vi "Main.vi"() -> ()   [LabVIEW 2025]
uses:
  Typedefs/MainState.ctl
  Typedefs/ConfigurationSettings.ctl
panel:
  in  "Reset":bool
  in  "Clear Data":bool
  in  "Configure":bool
  in  "Add Data":bool
  out "Waveform Chart":dbl[](graph)
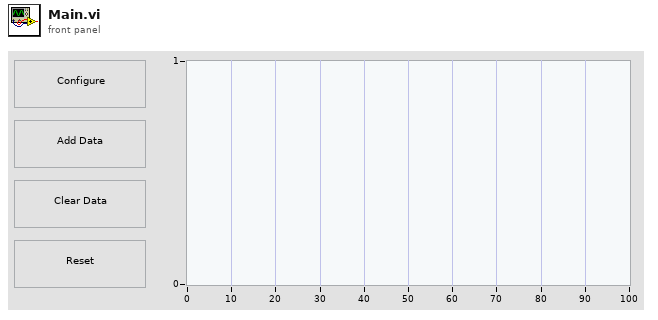
[diagram p1: front panel]
types:
  T1 = typedef "MainState.ctl" = enum16{"CONSTRUCT", "DESTRUCT", "WAITING_FOR_EVENT", "ADD_DATA", "CLEAR_DATA", "CONFIGURE", "RESET"}
  T2 = typedef "ConfigurationSettings.ctl" = cluster{"Plot.Line Width":u8, "Plot.Line Style":u8}
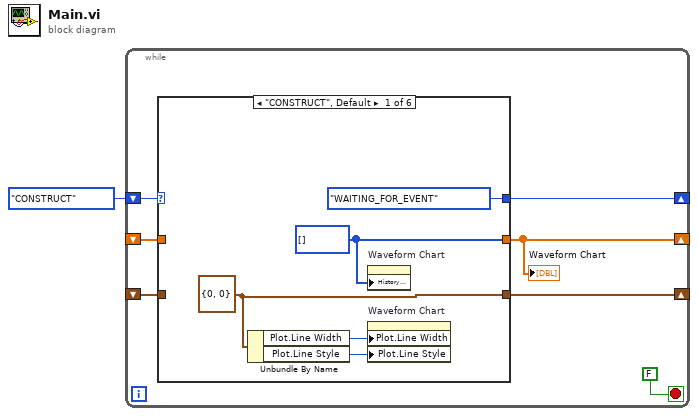
[diagram p0: block diagram]
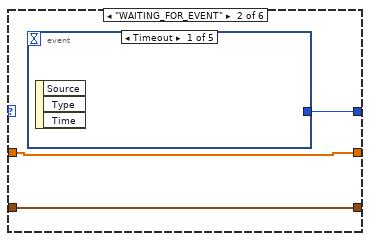
[diagram p2: hidden frame]
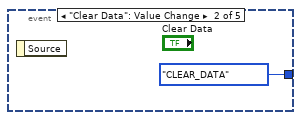
[diagram p3: hidden frame]
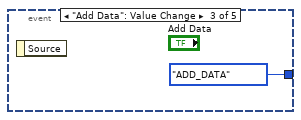
[diagram p4: hidden frame]
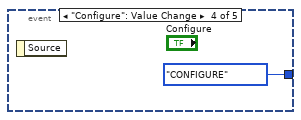
[diagram p5: hidden frame]
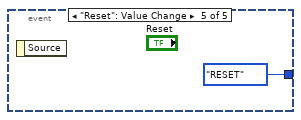
[diagram p6: hidden frame]
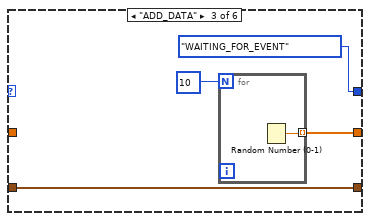
[diagram p7: hidden frame]
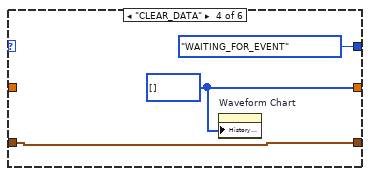
[diagram p8: hidden frame]
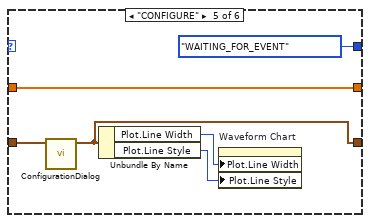
[diagram p9: hidden frame]
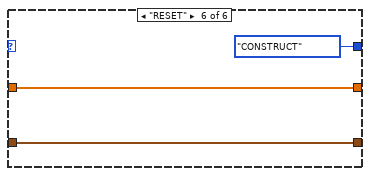
[diagram p10: hidden frame]
diagram:
  n1 = while {
    shift-right: [w6] -> _
    shift-left: MainState."CONSTRUCT" ("Main State") -> [w8]
    shift-right: [w7] -> _
    shift-left: _ -> [w5]
    shift-right: [w2] -> _
    shift-left: _ -> [w3]
    stop <- FALSE stop-if-true
    n2 = case shown="\"CONSTRUCT\", Default" w8 {
      tunnel: [w12 w15 w22 w27 w33 w36] -> w7
      tunnel: [MainState."WAITING_FOR_EVENT" ("Main State") w16 MainState."WAITING_FOR_EVENT" ("Main State") MainState."WAITING_FOR_EVENT" ("Main State") MainState."WAITING_FOR_EVENT" ("Main State") MainState."CONSTRUCT" ("Main State")] -> w6
      tunnel: w5 -> [_ w15 _ _ w33 w36]
      tunnel: w3 -> [_ w14 w21 w26 w32 w35]
      tunnel: [w11 w14 w21 w26 w31 w35] -> w2
      frame "CONSTRUCT", Default {
        w11 = T2 {"Plot.Line Width"=0, "Plot.Line Style"=0} ("ConfigurationSettings")
        w12 = i32[] []
        n3 = Unbundle By Name(w11) -> ("Plot.Line Width"=w10:u8, "Plot.Line Style"=w9:u8)
        n4 = property on="Waveform Chart" class="WFChart (strict)"("History Data"=w12) -> ()  [unwired: 2 in, 2 out]
        n5 = property on="Waveform Chart" class="WFChart (strict)"("Plot.Line Width"=w10, "Plot.Line Style"=w9) -> ()  [unwired: 2 in, 2 out]
      }
      frame "WAITING_FOR_EVENT" {
        n6 = event shown="[0] Timeout" {
          selector: _ -> [_ _ _ _ _]
          dyn-events: _ -> [_ _ _ _ _]
          timeout: _ -> [_ _ _ _ _]
          tunnel: [_ MainState."CLEAR_DATA" ("Main State") MainState."ADD_DATA" ("Main State") MainState."CONFIGURE" ("Main State") MainState."RESET" ("Main State")] -> w16
          event Timeout {
            n7 = event-data() -> ()  [unwired: 1 in, 3 out]
          }
          event "Clear Data": Value Change {
            n8 = event-data() -> ()  [unwired: 1 in, 1 out]
          }
          event "Add Data": Value Change {
            n9 = event-data() -> ()  [unwired: 1 in, 1 out]
          }
          event "Configure": Value Change {
            n10 = event-data() -> ()  [unwired: 1 in, 1 out]
          }
          event "Reset": Value Change {
            n11 = event-data() -> ()  [unwired: 1 in, 1 out]
          }
        }
      }
      frame "ADD_DATA" {
        n12 = for {
          N: 10 -> [_]
          tunnel: [w25] -> w22 mode=indexing
          n13 = Random Number (0-1)() -> (number: 0 to 1=w25:dbl)
        }
      }
      frame "CLEAR_DATA" {
        w27 = i32[] []
        n14 = property on="Waveform Chart" class="WFChart (strict)"("History Data"=w27) -> ()  [unwired: 2 in, 2 out]
      }
      frame "CONFIGURE" {
        n15 = call "ConfigurationDialog.vi"("Configuration Settings In"=w32) -> ("Configuration Settings Out"=w31:T2)  [unwired: 9 in, 1 out]
        n16 = Unbundle By Name(w31) -> ("Plot.Line Width"=w30:u8, "Plot.Line Style"=w29:u8)
        n17 = property on="Waveform Chart" class="WFChart (strict)"("Plot.Line Width"=w30, "Plot.Line Style"=w29) -> ()  [unwired: 2 in, 2 out]
      }
      frame "RESET" {
      }
    }
    "Waveform Chart" <- w7
  }
